vi "Close.vi"(8 "error in (no error)":errorcluster, 11 "reference in":refnum<class "Switch_Keysight_34934A.lvclass">) -> (0 "error out":errorcluster, 3 "reference in":refnum<class "Switch_Keysight_34934A.lvclass">)   [LabVIEW 2022 SP3, in "Switch_Keysight_34934A.lvlib" / "Switch_Keysight_34934A.lvclass"]
uses:
  Switch_Keysight_34934A.lvclass
  Components/SwitchBase.lvlibp/SwitchBase.lvclass
  Components/ViPER.lvlibp/ViPER.lvclass
  C:/Projects/Medulla/ViPER/Examples/Flux_Capacitor_Tester/Components/ViPER.lvlibp/ViPER.lvclass
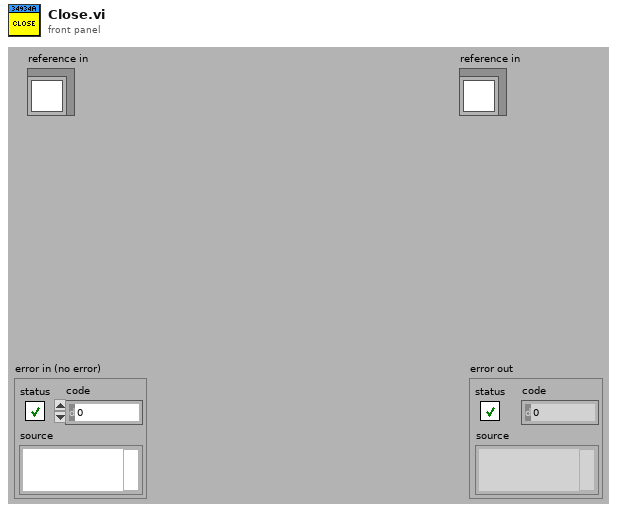
[diagram p1: front panel]
types:
  T1 = typedef "Switch_Keysight_34934A.lvlib/Switch_Keysight_34934A.lvclass/ObjectAttributes.ctl" = cluster{"Config":T2, "VISA ref":refnum<visa-resource-name>, "M1H":bool[][], "M2H":bool[][], "M1L":bool[][], "M2L":bool[][], "route":string, "State":bool[], "StateModBit":bool[], "UpdateEvent":refnum<user-event>}
  T2 = typedef "Switch_Keysight_34934A.lvlib/Switch_Keysight_34934A.lvclass/Config.ctl" = cluster{"VISA":refnum<visa-resource-name>, "Slot":i32, "SwitchMap":cluster{"Name":string, "Route":string[], "UnRoute":string[], "Description":string, "Group":string, "IsGroup":bool}[], "Sim":bool}
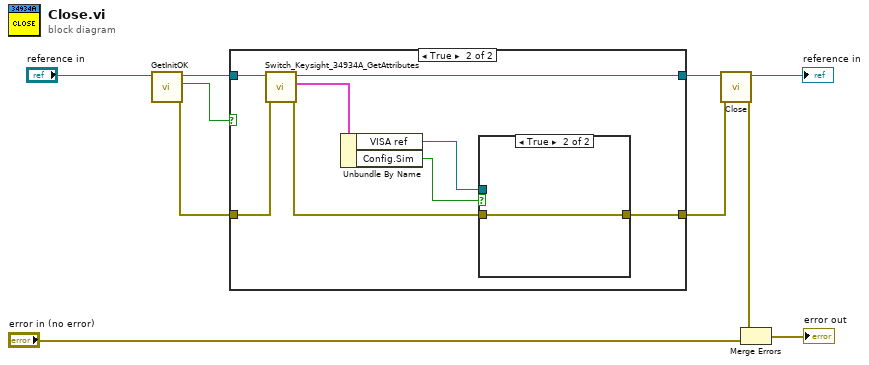
[diagram p0: block diagram]
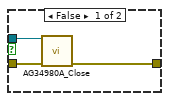
[diagram p3: hidden frame]
diagram:
  n1 = call "GetInitOK.vi"("reference in"="reference in") -> ("error out"=w4:errorcluster, "init_ok"=w5:bool, "reference out"=w6:refnum<class "Switch_Keysight_34934A.lvclass">)  [unwired: 8 in]
  n2 = case shown="True" w5 {
    tunnel: w4 -> [w12 w19]
    tunnel: [w12 w15] -> w7
    tunnel: w6 -> [w11 w20]
    tunnel: [w11 w18] -> w8
    frame False {
    }
    frame True {
      n3 = call "Switch_Keysight_34934A_GetAttributes.vi"("error in (no error)"=w19, "reference in"=w20) -> ("error out"=w16:errorcluster, "Data"=w17:T1, "reference out"=w18:refnum<class "Switch_Keysight_34934A.lvclass">)  [unwired: 6 in, 1 out]
      n4 = Unbundle By Name(w17) -> ("VISA ref"=w14:refnum<visa-resource-name>, "Config.Sim"=w13:bool)
      n5 = case shown="True" w13 {
        tunnel: w16 -> [w23 w24]
        tunnel: [w22 w24] -> w15
        tunnel: w14 -> [w21 _]
        frame False {
          n6 = call "AG34980A_Close.vi"("VISA resource name"=w21, "error in (no error)"=w23) -> ("error out"=w22:errorcluster)  [unwired: 13 in]
        }
        frame True {
        }
      }
    }
  }
  n7 = call-parent "Close.vi"("error in (no error)"=w7, "reference in"=w8) -> ("error out"=w3:errorcluster, "reference in"=→"reference in":refnum<class "Switch_Keysight_34934A.lvclass">)  [unwired: 8 in]
  n8 = Merge Errors(w3, "error in (no error)") -> (→"error out":errorcluster)
